vi "Handle.vi"(7 "Event Actor in":refnum<class "Event Actor.lvclass">, 11 "Teardown Event State in":refnum<class "Teardown Event State.lvclass">) -> (2 "Destroy?":bool, 5 "Event Actor out":refnum<class "Event Actor.lvclass">)   [LabVIEW 2021, in "jettl.lvlib" / "jettl Event Actor.lvlib" / "Teardown Event State.lvclass"]
uses:
  Teardown Event State.lvclass
  Actor/Event Actor/Event Actor.lvclass
  Teardown Event State.lvclass/Teardown Event State.ctl
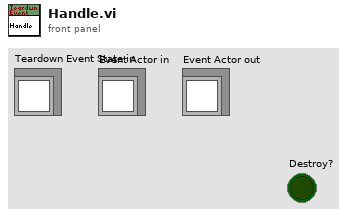
[diagram p1: front panel]
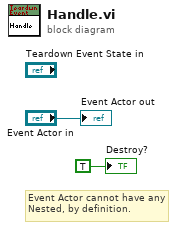
[diagram p0: block diagram]
diagram:
  # "Event Actor cannot have any Nested, by definition."
  "Destroy?" <- TRUE ("Destroy?")
  "Event Actor out" <- "Event Actor in"
